vi "Create Tags.vi"(8 "error in (no error)":errorcluster, 11 "Logger in.lvclass":refnum<class "Logger.lvclass">) -> (0 "error out":errorcluster, 3 "Logger out.lvclass":refnum<class "Logger.lvclass">)   [LabVIEW 2017, in "Logger.lvclass"]
uses:
  Logger.lvclass
  Logger.lvclass/Logger.ctl
  <vilib>/Skyline/Tag/Shared/typedefs/DataType.ctl
  <vilib>/Skyline/Tag/Wrapper/Wrapper AMQP_class/Open Tag AMQP.vi
  <vilib>/Skyline/Tag/Wrapper/Wrapper_class/NI Skyline Tag.lvclass
  <vilib>/Skyline/Tag/Shared/NI Skyline Tag.lvlib
  <vilib>/Skyline/Tag/Wrapper/Wrapper AMQP_class/NI Skyline Tag AMQP.lvclass
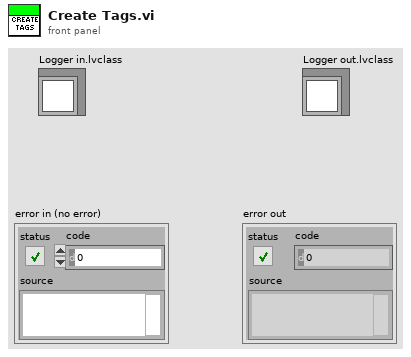
[diagram p1: front panel]
types:
  T1 = typedef "NI Skyline Tag.lvlib/DataType.ctl" = enum32{"Double", "Integer", "String"}
  T2 = cluster{"tag_updates":i32, "tag_publish_interval":i32, "tag_count":i32}
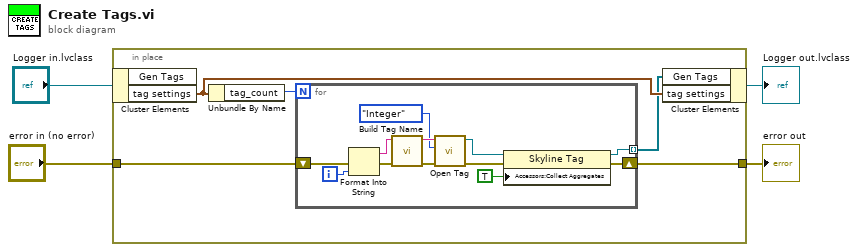
[diagram p0: block diagram]
diagram:
  n1 = in-place {
    in-place-border: "error in (no error)" -> [w7]
    in-place-border: [w6] -> w1
    n2 = in-place-cluster #1("Logger in.lvclass") -> ("tag settings"=w9:T2)  [unwired: 1 out]
    n3 = Unbundle By Name(w9) -> ("tag_count"=w8:i32)
    n4 = for {
      N: w8 -> [_]
      shift-right: [w11] -> w6
      shift-left: w7 -> [w16]
      tunnel: [w10] -> w5 mode=indexing
      i -> [w20]
      n5 = Format Into String(error in=w16, w20) -> (resulting string=w18:string, error out=w17:errorcluster)  [unwired: 2 in]
      n6 = call "Build Tag Name.vi"("error in (no error)"=w17, "Tag"=w18) -> ("error out"=w21:errorcluster, "System Tag"=w19:string)  [unwired: 8 in]
      n7 = call-poly <vilib>:"Open Tag.vi"("error in (no error)"=w21, "data type"=DataType."Integer" ("Data Type"), "path"=w19) -> ("error out"=w12:errorcluster, "tag out"=w14:refnum<class "NI Skyline Tag.lvclass">)  [unwired: 7 in]
      n8 = property class="Skyline Tag"(reference=w14, error in=w12, "Accessors:Collect Aggregates"=TRUE ("Collect Aggregates")) -> (reference out=w10:refnum<class "NI Skyline Tag.lvclass">, error out=w11:errorcluster)
    }
    n9 = in-place-cluster #1("Gen Tags"=w5, "tag settings"=w9) -> (→"Logger out.lvclass":refnum<class "Logger.lvclass">)
  }
  "error out" <- w1
